vi "Determine More Warnings.vi"(6 "Max Wind Speed":dbl, 7 "Current Wind Speed":dbl, 9 "Min Temp":dbl, 10 "Max Temp":dbl, 11 "Current Temp":dbl) -> (1 "Warning?":bool, 2 "Warning Text":string)   [LabVIEW 2014]
doc: "This VI is an exercise in the LabVIEW Core I course. In this exercise, you generate appropriate strings for Freeze, Heat Stroke, and High Wind warnings, and combinations of the warnings."
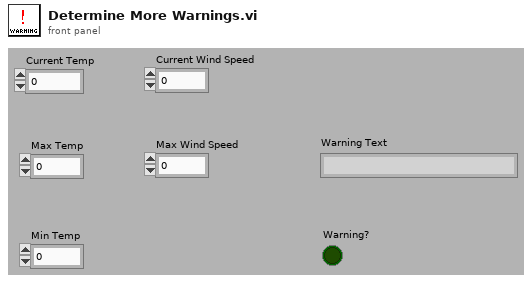
[diagram p1: front panel]
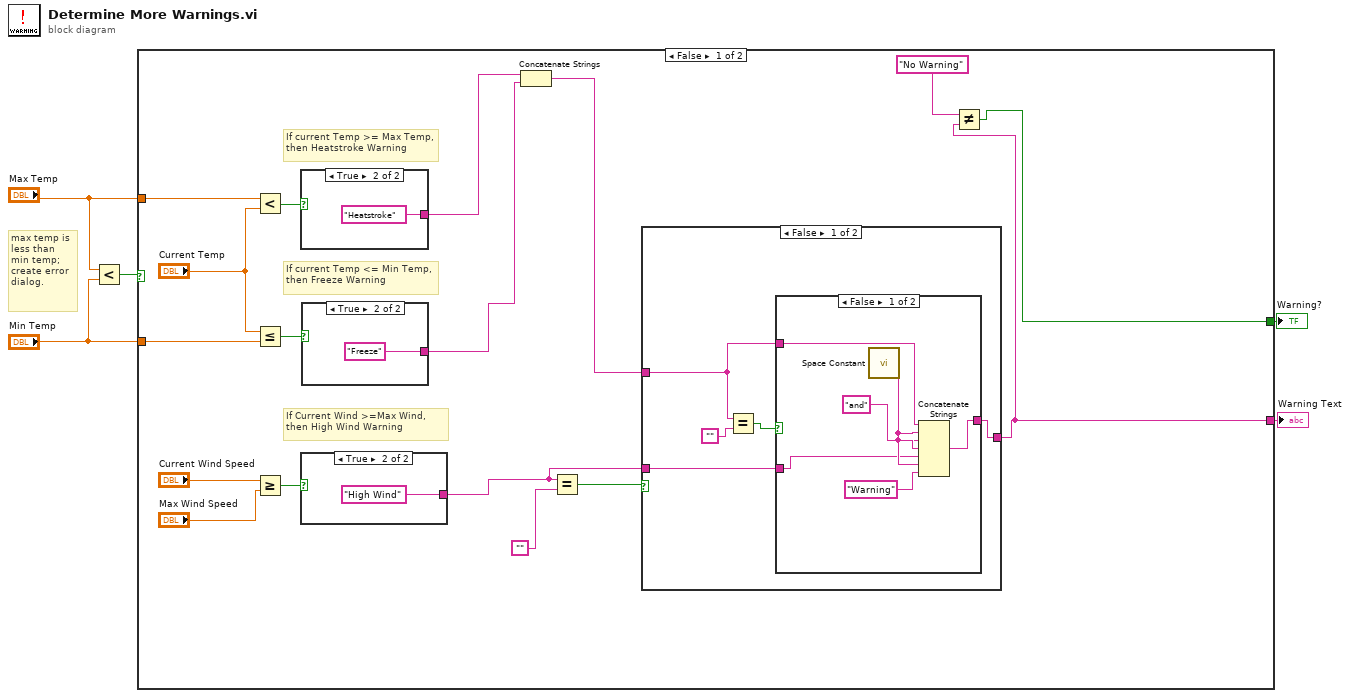
[diagram p0: block diagram]
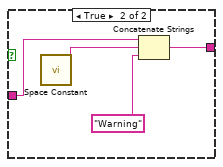
[diagram p2: hidden frame]
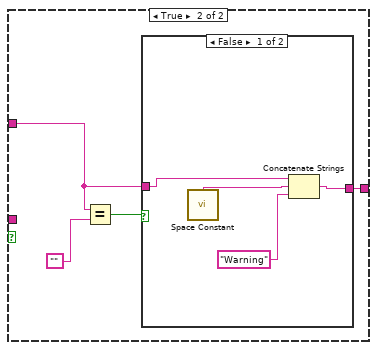
[diagram p3: hidden frame]
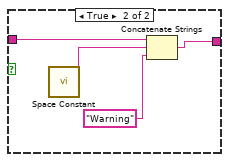
[diagram p4: hidden frame]
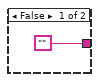
[diagram p5: hidden frame]
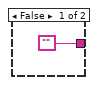
[diagram p6: hidden frame]
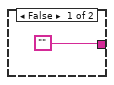
[diagram p7: hidden frame]
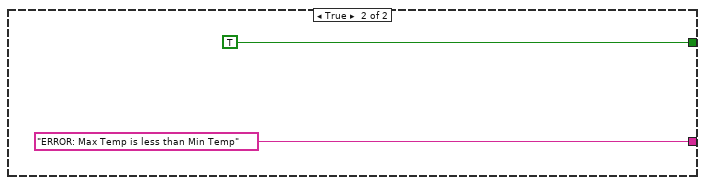
[diagram p8: hidden frame]
diagram:
  # "max temp is less than min temp; create error dialog."
  n1 = Less?(x="Max Temp", y="Min Temp") -> (x < y?=w1:bool)
  n2 = case shown="False" w1 {
    tunnel: [w7 TRUE] -> w5
    tunnel: [w6 "ERROR: Max Temp is less than Min Temp"] -> w4
    tunnel: "Max Temp" -> [w16 _]
    tunnel: "Min Temp" -> [w15 _]
    frame False {
      # "If Current Wind >=Max Wind, then High Wind Warning"
      # "If current Temp <= Min Temp, then Freeze Warning"
      # "If current Temp >= Max Temp, then Heatstroke Warning"
      n3 = Less?(x=w16, y="Current Temp") -> (x < y?=w20:bool)
      n4 = Less Or Equal?(x="Current Temp", y=w15) -> (x <= y?=w22:bool)
      n5 = Greater Or Equal?(x="Current Wind Speed", y="Max Wind Speed") -> (x >= y?=w17:bool)
      n6 = case shown="True" w20 {
        tunnel: ["" "Heatstroke"] -> w8
        frame False {
        }
        frame True {
        }
      }
      n7 = case shown="True" w17 {
        tunnel: ["" "High Wind"] -> w10
        frame False {
        }
        frame True {
        }
      }
      n8 = case shown="True" w22 {
        tunnel: ["" "Freeze"] -> w9
        frame False {
        }
        frame True {
        }
      }
      n9 = Concatenate Strings(w8, w9) -> (w12:string)
      n10 = Equal?(x=w10, y="") -> (x = y?=w14:bool)
      n11 = case shown="False" w14 {
        tunnel: w12 -> [w24 w41]
        tunnel: w10 -> [w25 _]
        tunnel: [w23 w39] -> w6
        frame False {
          n12 = Equal?(x=w24, y="") -> (x = y?=w27:bool)
          n13 = case shown="False" w27 {
            tunnel: w25 -> [w30 w37]
            tunnel: w24 -> [w32 _]
            tunnel: [w28 w34] -> w23
            frame False {
              n14 = call <vilib>:"Space Constant.vi"() -> ("String"=w33:string)
              n15 = Concatenate Strings(w32, w33, "and", w33, w30, w33, "Warning") -> (w28:string)
            }
            frame True {
              n16 = call <vilib>:"Space Constant.vi"() -> ("String"=w36:string)
              n17 = Concatenate Strings(w37, w36, "Warning") -> (w34:string)
            }
          }
        }
        frame True {
          n18 = Equal?(x=w41, y="") -> (x = y?=w40:bool)
          n19 = case shown="False" w40 {
            tunnel: w41 -> [w43 w49]
            tunnel: [w45 w46] -> w39
            frame False {
              n20 = call <vilib>:"Space Constant.vi"() -> ("String"=w44:string)
              n21 = Concatenate Strings(w43, w44, "Warning") -> (w45:string)
            }
            frame True {
              n22 = call <vilib>:"Space Constant.vi"() -> ("String"=w48:string)
              n23 = Concatenate Strings(w49, w48, "Warning") -> (w46:string)
            }
          }
        }
      }
      n24 = Not Equal?(x="No Warning", y=w6) -> (x != y?=w7:bool)
    }
    frame True {
    }
  }
  "Warning Text" <- w4
  "Warning?" <- w5
